vi "getChannelAddresses.vi"(8 "error in (no error)":errorcluster, 11 "ScriptEventList in":refnum<class "ScriptEventList.lvclass">) -> (0 "error out":errorcluster, 2 "ChannelAddresses":string[](array[string]), 3 "ScriptEventList out":refnum<class "ScriptEventList.lvclass">)   [LabVIEW 2009, in "Tools.lvlib" / "Scripting.lvlib" / "ScriptEventList.lvclass"]
uses:
  ScriptEventList.lvclass
  ScriptEventList.lvclass/ScriptEventList.ctl
  ScriptEvent.lvclass
  DatabaseHelpers/Database Objects/Channel/Channel.lvclass
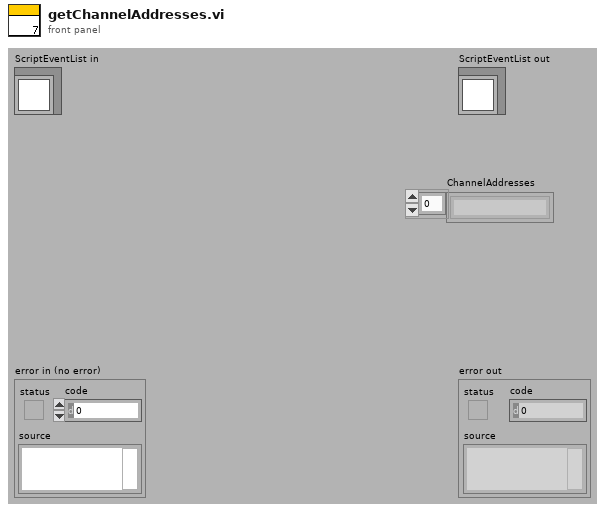
[diagram p1: front panel]
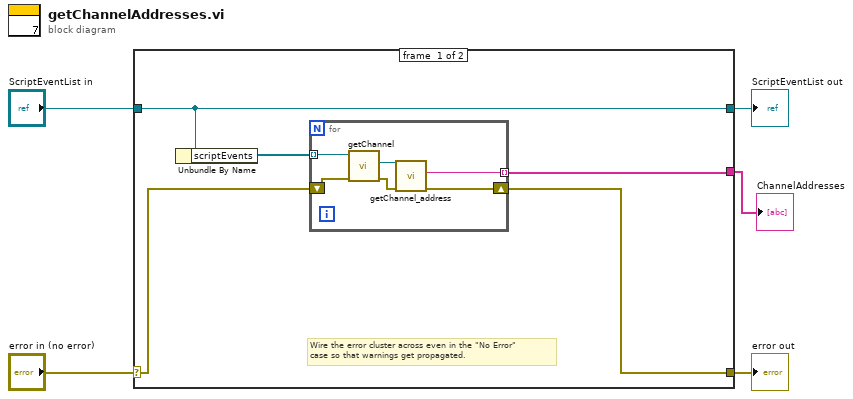
[diagram p0: block diagram]
diagram:
  n1 = case shown="No Error" "error in (no error)" {
    selector: "error in (no error)" -> [w7 w18]
    tunnel: [w6 w18] -> w4
    tunnel: [w10 w17] -> w2
    tunnel: "ScriptEventList in" -> [w10 w17]
    tunnel: [w8 _] -> w1
    frame #0 {
      # "Wire the error cluster across even in the \"No Error\"\ncase so that warnings get propagated."
      n2 = Unbundle By Name(w10) -> ("scriptEvents"=w9:refnum<class "ScriptEvent.lvclass">[])
      n3 = for {
        tunnel: w9 -> [w14] mode=indexing
        shift-right: [w12] -> w6
        shift-left: w7 -> [w13]
        tunnel: [w11] -> w8 mode=indexing
        n4 = call-dynamic "getChannel.vi"("error in (no error)"=w13, "ScriptEvent.lvclass in"=w14) -> ("error out"=w15:errorcluster, "Channel.lvclass"=w16:refnum<class "Channel.lvclass">)  [unwired: 7 in, 1 out]
        n5 = call "getChannel_address.vi"("error in (no error)"=w15, "Channel.lvclass in"=w16) -> ("error out"=w12:errorcluster, "channel_address"=w11:string)  [unwired: 7 in, 1 out]
      }
    }
    frame #1 {
    }
  }
  "error out" <- w4
  "ScriptEventList out" <- w2
  "ChannelAddresses" <- w1
